vi "Manipulator_Log_(string).vi"() -> ()   [LabVIEW 2013]
panel:
  in  "Manipulator Log":string
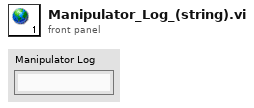
[diagram p1: front panel]
diagram:
